vi "Create All Message Queues.vi"(8 "error in (no error)":errorcluster) -> (0 "error out":errorcluster, 3 "Message Queues out":T1)   [LabVIEW 2013, in "Message Queue.lvlib"]
doc: "This VI creates and initializes all the message queues for your application. If your application requires more than one message queue, right-click the \"Message Queues\" constant above and select Open Type Def. Add the new Message Queue(s) to the type definition, then initialize them in this VI."
uses:
  Message Queue.lvlib
  All Message Queues.ctl
  Message Cluster.ctl
  Enqueue Message (Single).vi
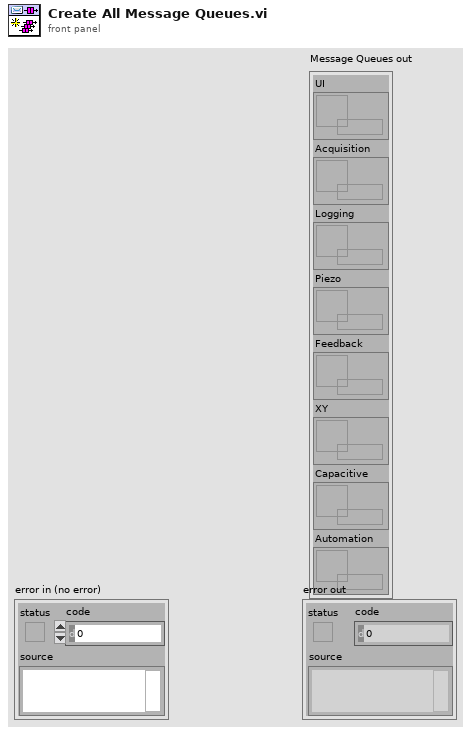
[diagram p1: front panel]
types:
  T1 = typedef "Message Queue.lvlib/All Message Queues.ctl" = cluster{"UI":refnum<queue>, "Acquisition":refnum<queue>, "Logging":refnum<queue>, "Piezo":refnum<queue>, "Feedback":refnum<queue>, "XY":refnum<queue>, "Capacitive":refnum<queue>, "Automation":refnum<queue>}
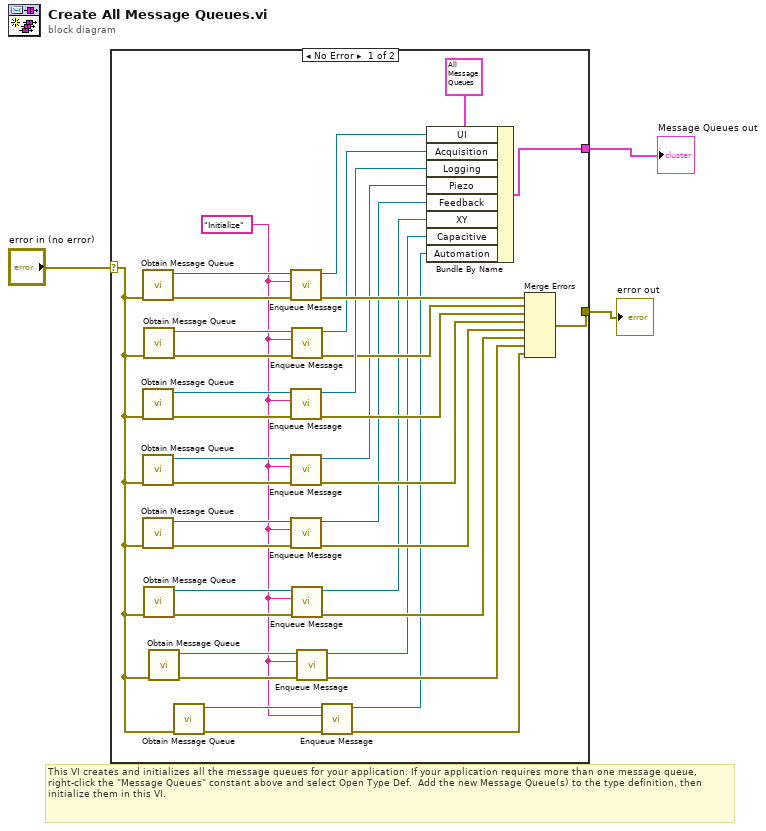
[diagram p0: block diagram]
diagram:
  # "This VI creates and initializes all the message queues for your application. If your application requires more than one message queue, right-click the \"Message Queues\" constant above and select Open Type Def.  Add the new Message Queue(s) to the type definition, then initialize them in this VI."
  n1 = case shown="No Error" "error in (no error)" {
    selector: "error in (no error)" -> [w7 w41]
    tunnel: [w28 w41] -> w3
    tunnel: [w38 _] -> w2
    frame No Error {
      w5 = "Initialize" ("Message")
      n2 = call "Obtain Message Queue.vi"("error in (no error)"=w7) -> ("error out"=w37:errorcluster, "Message Queue"=w36:refnum<queue>)  [unwired: 9 in]
      n3 = call "Obtain Message Queue.vi"("error in (no error)"=w7) -> ("error out"=w33:errorcluster, "Message Queue"=w32:refnum<queue>)  [unwired: 9 in]
      n4 = call "Obtain Message Queue.vi"("error in (no error)"=w7) -> ("error out"=w25:errorcluster, "Message Queue"=w24:refnum<queue>)  [unwired: 9 in]
      n5 = call "Obtain Message Queue.vi"("error in (no error)"=w7) -> ("error out"=w21:errorcluster, "Message Queue"=w20:refnum<queue>)  [unwired: 9 in]
      n6 = call "Obtain Message Queue.vi"("error in (no error)"=w7) -> ("error out"=w34:errorcluster, "Message Queue"=w35:refnum<queue>)  [unwired: 9 in]
      n7 = call "Obtain Message Queue.vi"("error in (no error)"=w7) -> ("error out"=w17:errorcluster, "Message Queue"=w16:refnum<queue>)  [unwired: 9 in]
      n8 = call "Obtain Message Queue.vi"("error in (no error)"=w7) -> ("error out"=w13:errorcluster, "Message Queue"=w11:refnum<queue>)  [unwired: 9 in]
      n9 = call "Obtain Message Queue.vi"("error in (no error)"=w7) -> ("error out"=w9:errorcluster, "Message Queue"=w8:refnum<queue>)  [unwired: 9 in]
      n10 = call-poly "Enqueue Message.vi"("error in (no error)"=w37, "Message"=w5, "Message Queue"=w36) -> ("error out"=w40:errorcluster, "dup Message Queue"=w31:refnum<queue>)  [unwired: 7 in]
      n11 = call-poly "Enqueue Message.vi"("error in (no error)"=w33, "Message"=w5, "Message Queue"=w32) -> ("error out"=w26:errorcluster, "dup Message Queue"=w29:refnum<queue>)  [unwired: 7 in]
      n12 = call-poly "Enqueue Message.vi"("error in (no error)"=w25, "Message"=w5, "Message Queue"=w24) -> ("error out"=w22:errorcluster, "dup Message Queue"=w23:refnum<queue>)  [unwired: 7 in]
      n13 = call-poly "Enqueue Message.vi"("error in (no error)"=w21, "Message"=w5, "Message Queue"=w20) -> ("error out"=w18:errorcluster, "dup Message Queue"=w19:refnum<queue>)  [unwired: 7 in]
      n14 = call-poly "Enqueue Message.vi"("error in (no error)"=w34, "Message"=w5, "Message Queue"=w35) -> ("error out"=w27:errorcluster, "dup Message Queue"=w30:refnum<queue>)  [unwired: 7 in]
      n15 = call-poly "Enqueue Message.vi"("error in (no error)"=w17, "Message"=w5, "Message Queue"=w16) -> ("error out"=w14:errorcluster, "dup Message Queue"=w15:refnum<queue>)  [unwired: 7 in]
      n16 = call-poly "Enqueue Message.vi"("error in (no error)"=w13, "Message"=w5, "Message Queue"=w11) -> ("error out"=w12:errorcluster, "dup Message Queue"=w10:refnum<queue>)  [unwired: 7 in]
      n17 = call-poly "Enqueue Message.vi"("error in (no error)"=w9, "Message"=w5, "Message Queue"=w8) -> ("error out"=w6:errorcluster, "dup Message Queue"=w4:refnum<queue>)  [unwired: 7 in]
      n18 = Bundle By Name(cluster=T1 {"UI"=refnum, "Acquisition"=refnum, "Logging"=refnum, "Piezo"=refnum, "Feedback"=refnum, "XY"=refnum, "Capacitive"=refnum, "Automation"=refnum} ("Message Queues"), "UI"=w31, "Acquisition"=w30, "Logging"=w29, "Piezo"=w23, "Feedback"=w19, "XY"=w15, "Capacitive"=w10, "Automation"=w4) -> (w38:T1)
      n19 = Merge Errors(w40, w27, w26, w22, w18, w14, w12, w6) -> (w28:errorcluster)
    }
    frame Error {
    }
  }
  "Message Queues out" <- w2
  "error out" <- w3
